vi "Auto Drive.vi"(0 "Drive Dev Ref in":T5={"DevStatus"={"status"=FALSE, "code"=0, "source"=""}, "Motors[]"=[{"DeviceStatus"={"status"=FALSE, "code"=0, "source"=""}, "Type"=enum."CAN", "PWM"={"PWM Channel"=enum."PWM 1", "DeadBand"={"Name"="", "maxPositivePwm"=0, "minPositivePwm"=0, "centerPwm"=0, "maxNegativePwm"=0, "minNegativePwm"=0, "angularRange"=0}}, "CAN"={"Device Number"=1, "SetOutput VI Ref"=variant(refnum<vi> refnum), "GetOutput VI Ref"=variant(refnum<vi> refnum), "Enable VI Ref"=variant(refnum<vi> refnum), "Disable VI Ref"=variant(refnum<vi> refnum), "Data"=variant(cluster{"Library":path, "handle":u64, "Control Mode":u16, "UsageFrame":u32, "RefNumName":string, "arbID":u32} {"Library"=path "libCTRE_PhoenixCCI.so", "handle"=21905672, "Control Mode"=0, "UsageFrame"=0, "RefNumName"="", "arbID"=33816577})}, "Invert"=TRUE, "DIO PWM"={"PWM \"Enable\" Channel"=enum."Invalid", "DIOChannel"=enum."Invalid", "PWM Rate"=0.0}}, {"DeviceStatus"={"status"=FALSE, "code"=0, "source"=""}, "Type"=enum."CAN", "PWM"={"PWM Channel"=enum."PWM 1", "DeadBand"={"Name"="", "maxPositivePwm"=0, "minPositivePwm"=0, "centerPwm"=0, "maxNegativePwm"=0, "minNegativePwm"=0, "angularRange"=0}}, "CAN"={"Device Number"=13, "SetOutput VI Ref"=variant(refnum<vi> refnum), "GetOutput VI Ref"=variant(refnum<vi> refnum), "Enable VI Ref"=variant(refnum<vi> refnum), "Disable VI Ref"=variant(refnum<vi> refnum), "Data"=variant(cluster{"Library":path, "handle":u64, "Control Mode":u16, "UsageFrame":u32, "RefNumName":string, "arbID":u32} {"Library"=path "libCTRE_PhoenixCCI.so", "handle"=21919480, "Control Mode"=0, "UsageFrame"=0, "RefNumName"="", "arbID"=33816589})}, "Invert"=FALSE, "DIO PWM"={"PWM \"Enable\" Channel"=enum."Invalid", "DIOChannel"=enum."Invalid", "PWM Rate"=0.0}}], "Square Inputs"=FALSE, "Max Output"=1.0}, 5 "Gyro Dev Ref in":T11={"DevStatus"={"status"=FALSE, "code"=0, "source"=""}, "Analog Channel"=enum."AI 1", "Gain (VoltsPerDegree/Second)"=0.0, "Gyro Type"=enum."XRS450", "Handle"=8, "SPI Bus"=enum."SPI On-Board, CS0", "Device Found"=TRUE, "Sample Rate"=2000.0, "Calibrate On Open"=FALSE, "Offset"=0.21654062499999974} {"Sample Rate" min=0.25 max=100.0 step=0.25}, 9 "Encoder Dev Ref in":T1={"DevStatus"={"status"=FALSE, "code"=0, "source"=""}, "EncoderIndex"=enum."Enc 0", "CounterIndex"=enum."Invalid", "DistancePerCount"=1.0, "Decoding Type"=enum."4x"}, 12 "X setpoint":dbl=10.0 format="%#_13g", 14 "Y setpoint":dbl=-60.0 format="%.2f") -> (4 "Drive Dev Ref out":T5={"DevStatus"={"status"=FALSE, "code"=0, "source"=""}, "Motors[]"=[{"DeviceStatus"={"status"=FALSE, "code"=0, "source"=""}, "Type"=enum."CAN", "PWM"={"PWM Channel"=enum."PWM 1", "DeadBand"={"Name"="", "maxPositivePwm"=0, "minPositivePwm"=0, "centerPwm"=0, "maxNegativePwm"=0, "minNegativePwm"=0, "angularRange"=0}}, "CAN"={"Device Number"=1, "SetOutput VI Ref"=variant(refnum<vi> refnum), "GetOutput VI Ref"=variant(refnum<vi> refnum), "Enable VI Ref"=variant(refnum<vi> refnum), "Disable VI Ref"=variant(refnum<vi> refnum), "Data"=variant(cluster{"Library":path, "handle":u64, "Control Mode":u16, "UsageFrame":u32, "RefNumName":string, "arbID":u32} {"Library"=path "libCTRE_PhoenixCCI.so", "handle"=21905672, "Control Mode"=0, "UsageFrame"=0, "RefNumName"="", "arbID"=33816577})}, "Invert"=TRUE, "DIO PWM"={"PWM \"Enable\" Channel"=enum."Invalid", "DIOChannel"=enum."Invalid", "PWM Rate"=0.0}}, {"DeviceStatus"={"status"=FALSE, "code"=0, "source"=""}, "Type"=enum."CAN", "PWM"={"PWM Channel"=enum."PWM 1", "DeadBand"={"Name"="", "maxPositivePwm"=0, "minPositivePwm"=0, "centerPwm"=0, "maxNegativePwm"=0, "minNegativePwm"=0, "angularRange"=0}}, "CAN"={"Device Number"=13, "SetOutput VI Ref"=variant(refnum<vi> refnum), "GetOutput VI Ref"=variant(refnum<vi> refnum), "Enable VI Ref"=variant(refnum<vi> refnum), "Disable VI Ref"=variant(refnum<vi> refnum), "Data"=variant(cluster{"Library":path, "handle":u64, "Control Mode":u16, "UsageFrame":u32, "RefNumName":string, "arbID":u32} {"Library"=path "libCTRE_PhoenixCCI.so", "handle"=21919480, "Control Mode"=0, "UsageFrame"=0, "RefNumName"="", "arbID"=33816589})}, "Invert"=FALSE, "DIO PWM"={"PWM \"Enable\" Channel"=enum."Invalid", "DIOChannel"=enum."Invalid", "PWM Rate"=0.0}}], "Square Inputs"=FALSE, "Max Output"=1.0}, 6 "Gyro Dev Ref out":T11={"DevStatus"={"status"=FALSE, "code"=0, "source"=""}, "Analog Channel"=enum."AI 1", "Gain (VoltsPerDegree/Second)"=0.0, "Gyro Type"=enum."XRS450", "Handle"=8, "SPI Bus"=enum."SPI On-Board, CS0", "Device Found"=TRUE, "Sample Rate"=2000.0, "Calibrate On Open"=FALSE, "Offset"=0.21654062499999974} {"Sample Rate" min=0.25 max=100.0 step=0.25}, 8 "last y value":dbl=0.16038021312985137, 10 "Encoder Dev Ref out":T1={"DevStatus"={"status"=FALSE, "code"=0, "source"=""}, "EncoderIndex"=enum."Enc 0", "CounterIndex"=enum."Invalid", "DistancePerCount"=1.0, "Decoding Type"=enum."4x"}, 15 "In Range?":bool=TRUE)   [LabVIEW 2017]
uses:
  <vilib>/Rock Robotics/WPI/RobotDrive/WPI_RobotDriveDevRef.ctl
  <vilib>/Rock Robotics/WPI/MotorControl/WPI_MotorControlDeviceRef.ctl
  <vilib>/Rock Robotics/WPI/MotorControl/WPI_MotorControlType.ctl
  <vilib>/Rock Robotics/SystemInterfaces/DIO/FPGA_DIOPWMChannel.ctl
  <vilib>/Rock Robotics/WPI/PWM/WPI_PWMDeadband.ctl
  <vilib>/Rock Robotics/SystemInterfaces/DIO/FPGA_DIOChannel.ctl
  <vilib>/Rock Robotics/WPI/Gyro/WPI_GyroDevRef.ctl
  <vilib>/Rock Robotics/SystemInterfaces/AI/FPGA_AIChannel.ctl
  <vilib>/Rock Robotics/SystemInterfaces/spilib/spi_bus.ctl
  <vilib>/Rock Robotics/WPI/Encoder/WPI_EncoderDevRef.ctl
  <vilib>/Rock Robotics/SystemInterfaces/Encoder/FPGA_EncoderIdx.ctl
  <vilib>/Rock Robotics/SystemInterfaces/Counter/FPGA_CounterCtrSystemIndex.ctl
  <vilib>/Rock Robotics/WPI/Encoder/WPI_EncoderType.ctl
  <vilib>/Rock Robotics/WPI/RobotDrive/WPI_RobotDriveArcadeDrive_Standard(NoSaturation).vi
panel:
  in  "Drive Stop Tolerance":dbl=10.0
  in  "Y Max Speed":dbl=0.8999999999999999
  in  "Slowdown Range":dbl=45.0
  in  "Turn P Multiplier":dbl=0.03
  # "turn p 0.03"
  # "degrees"
  # "x set 10"
  # "inches"
  # "y set -60.00"
  # "slowdown 60"
  # "inches"
  # "Y max 0.9"
  # "inches"
  # "Drive tol. 10"
  # "Analog"
  # "XRS"
  # "Analog"
  # "XRS"
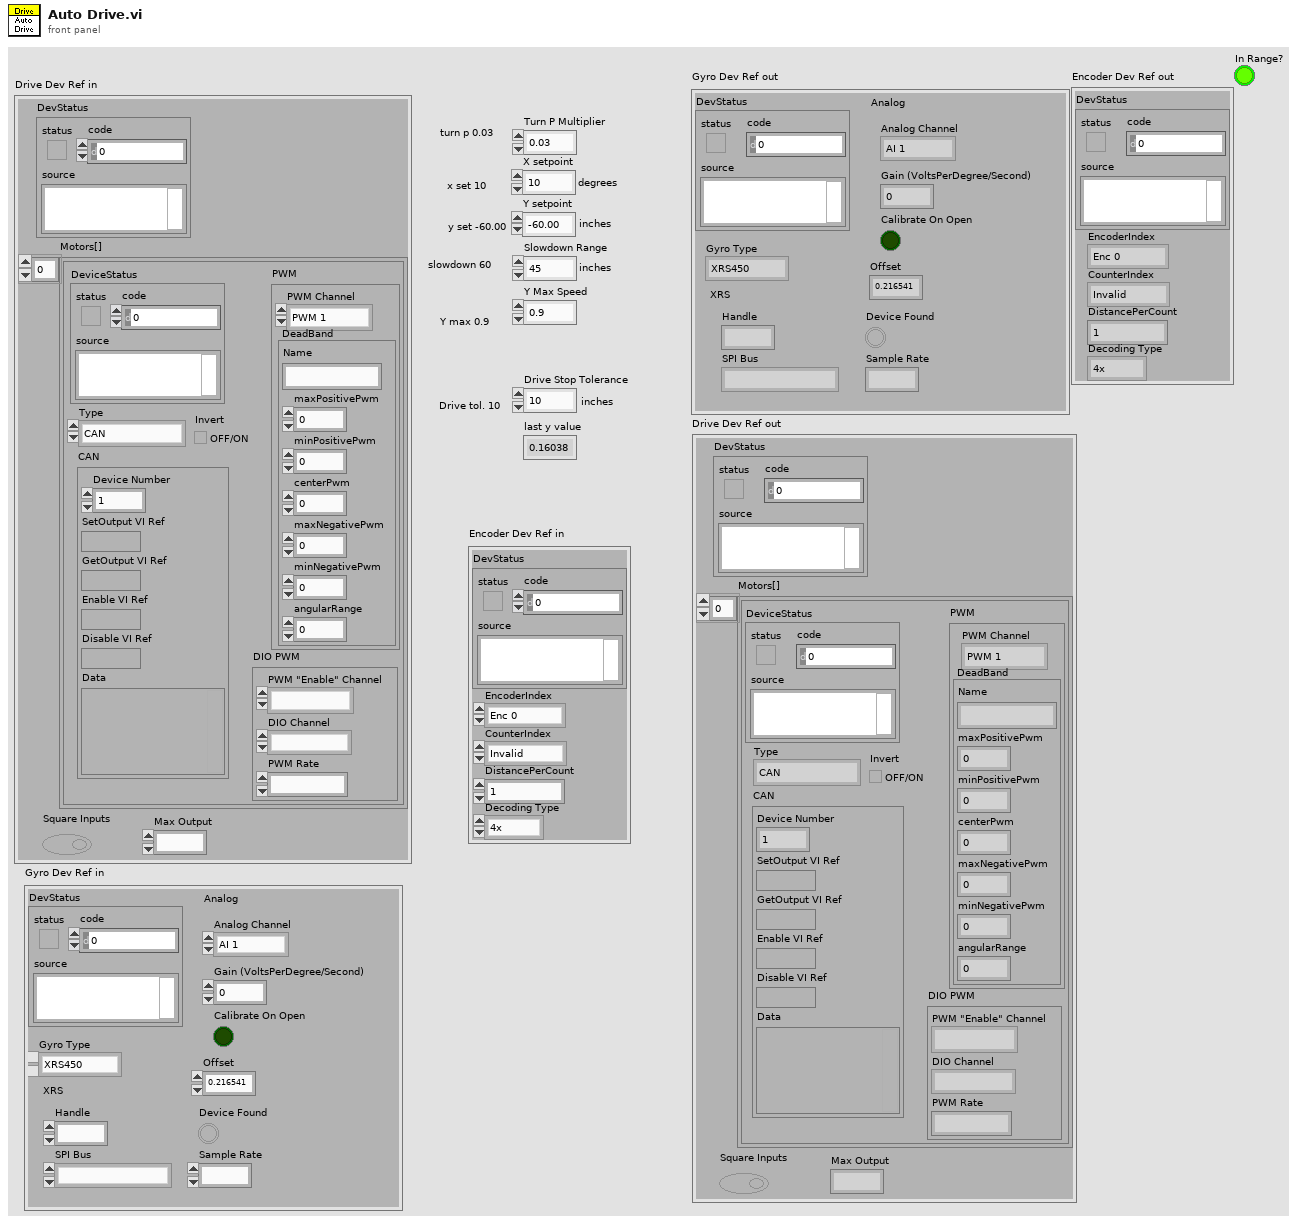
[diagram p1: front panel]
types:
  T1 = typedef "WPI_EncoderDevRef.ctl" = cluster{"DevStatus":errorcluster, "EncoderIndex":T2, "CounterIndex":T3, "DistancePerCount":dbl, "Decoding Type":T4}
  T2 = typedef "FPGA_EncoderIdx.ctl" = enum8{"Enc 0", "Enc 1", "Enc 2", "Enc 3", "Enc 4", "Enc 5", "Enc 6", "Enc 7", "Invalid"}
  T3 = typedef "FPGA_CounterCtrSystemIndex.ctl" = enum8{"Ctr 0", "Ctr 1", "Ctr 2", "Ctr 3", "Ctr 4", "Ctr 5", "Ctr 6", "Ctr 7", "Invalid"}
  T4 = typedef "WPI_EncoderType.ctl" = enum16{"1x", "2x", "4x"}
  T5 = typedef "WPI_RobotDriveDevRef.ctl" = cluster{"DevStatus":errorcluster, "Motors[]":T6[], "Square Inputs":bool, "Max Output":dbl}
  T6 = typedef "WPI_MotorControlDeviceRef.ctl" = cluster{"DeviceStatus":errorcluster, "Type":T7, "PWM":cluster{"PWM Channel":T8, "DeadBand":T9}, "CAN":cluster{"Device Number":u8, "SetOutput VI Ref":variant, "GetOutput VI Ref":variant, "Enable VI Ref":variant, "Disable VI Ref":variant, "Data":variant}, "Invert":bool, "DIO PWM":cluster{"PWM \"Enable\" Channel":T8, "DIOChannel":T10, "PWM Rate":dbl}}
  T7 = typedef "WPI_MotorControlType.ctl" = enum16{"PWM", "CAN", "DIO PWM"}
  T8 = typedef "FPGA_DIOPWMChannel.ctl" = enum8{"PWM 0", "PWM 1", "PWM 2", "PWM 3", "PWM 4", "PWM 5", "PWM 6", "PWM 7", "PWM 8", "PWM 9", "PWM MXP 0", "PWM MXP 1", "PWM MXP 2", "PWM MXP 3", "PWM MXP 4", "PWM MXP 5", "PWM MXP 6", "PWM MXP 7", "PWM MXP 8", "PWM MXP 9", "Invalid"}
  T9 = typedef "WPI_PWMDeadband.ctl" = cluster{"Name":string, "maxPositivePwm":i32, "minPositivePwm":i32, "centerPwm":i32, "maxNegativePwm":i32, "minNegativePwm":i32, "angularRange":u16}
  T10 = typedef "FPGA_DIOChannel.ctl" = enum8{"DIO 0", "DIO 1", "DIO 2", "DIO 3", "DIO 4", "DIO 5", "DIO 6", "DIO 7", "DIO 8", "DIO 9", "DIO MXP 0", "DIO MXP 1", "DIO MXP 2", "DIO MXP 3", "DIO MXP 4", "DIO MXP 5", "DIO MXP 6", "DIO MXP 7", "DIO MXP 8", "DIO MXP 9", "DIO MXP 10", "DIO MXP 11", "DIO MXP 12", "DIO MXP 13", "DIO MXP 14", "DIO MXP 15", "SPI Port CS1", "SPI Port CS2", "SPI Port CS3", "SPI Port MISO", "SPI Port MOSI", "Invalid"}
  T11 = typedef "WPI_GyroDevRef.ctl" = cluster{"DevStatus":errorcluster, "Analog Channel":T12, "Gain (VoltsPerDegree/Second)":dbl, "Gyro Type":enum16{"Analog", "XRS450"}, "Handle":i32, "SPI Bus":T13, "Device Found":bool, "Sample Rate":dbl, "Calibrate On Open":bool, "Offset":dbl}
  T12 = typedef "FPGA_AIChannel.ctl" = enum8{"AI 0", "AI 1", "AI 2", "AI 3", "AI MXP 0", "AI MXP 1", "AI MXP 2", "AI MXP 3", "Invalid"}
  T13 = typedef "spi_bus.ctl" = enum16{"SPI On-Board, CS0", "SPI On-Board, CS1", "SPI On-Board, CS2", "SPI On-Board, CS3", "SPI MXP", "Invalid"}
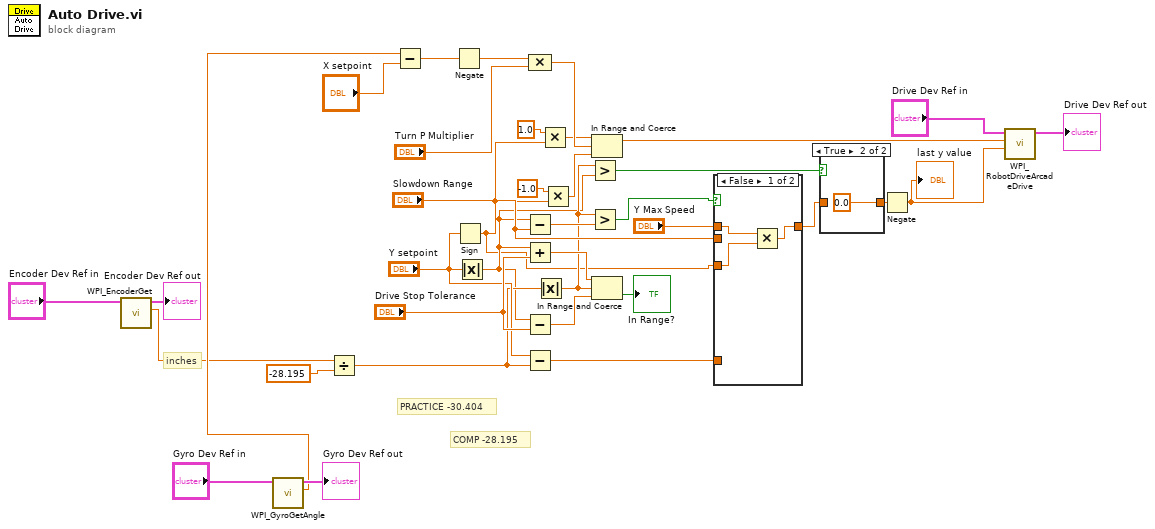
[diagram p0: block diagram]
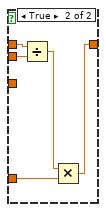
[diagram p3: hidden frame]
diagram:
  # "COMP -28.195"
  # "PRACTICE -30.404"
  # "inches"
  n1 = call <vilib>:"WPI_EncoderGet.vi"("EncoderDevRef"="Encoder Dev Ref in") -> ("Distance"=w16:dbl, "EncoderDevRef"=→"Encoder Dev Ref out":T1)  [unwired: 5 in, 4 out]
  n2 = call <vilib>:"WPI_GyroGetAngle.vi"("GyroDevRef"="Gyro Dev Ref in") -> ("Angle"=w31:dbl, "GyroDevRef"=→"Gyro Dev Ref out":T11)  [unwired: 6 in, 3 out]
  n3 = Divide(x=w16, y=-28.195) -> (x/y=w11:dbl)
  n4 = Subtract(x=w31, y="X setpoint") -> (x-y=w23:dbl)
  n5 = Negate(x=w23) -> (-x=w24:dbl)
  n6 = Sign(1:"Y setpoint") -> (0:w3:dbl)
  n7 = Absolute Value(x="Y setpoint") -> (abs(x)=w7:dbl)
  n8 = Subtract(x=w7, y="Slowdown Range") -> (x-y=w10:dbl)
  n9 = Add(x=w7, y="Drive Stop Tolerance") -> (x+y=w26:dbl)
  n10 = Subtract(x=w7, y="Drive Stop Tolerance") -> (x-y=w27:dbl)
  n11 = Subtract(x="Y setpoint", y=w11) -> (x-y=w12:dbl)
  n12 = Compound Arithmetic op=MULTIPLY(w24, "Turn P Multiplier") -> (w22:dbl)
  n13 = Absolute Value(x=w11) -> (abs(x)=w8:dbl)
  n14 = Multiply(x=1.0 ("upper limit"), y=w3) -> (x*y=w19:dbl)
  n15 = Multiply(x=-1.0 ("lower limit"), y=w3) -> (x*y=w17:dbl)
  n16 = Greater?(x=w8, y=w7) -> (0:w6:bool)
  n17 = Greater?(x=w8, y=w10) -> (0:w15:bool)
  n18 = In Range and Coerce(upper limit=w19, x=w22, lower limit=w17) -> (coerced(x)=w14:dbl)  [unwired: 1 out]
  n19 = In Range and Coerce(upper limit=w26, x=w8, lower limit=w27) -> (In Range?=→"In Range?":bool)  [unwired: 1 out]
  n20 = case shown="False" w15 {
    tunnel: [w38 w44] -> w5
    tunnel: "Y Max Speed" -> [w40 w43]
    tunnel: w12 -> [_ w45]
    tunnel: "Slowdown Range" -> [_ w42]
    tunnel: w3 -> [w39 _]
    frame False {
      n21 = Multiply(x=w40, y=w39) -> (x*y=w38:dbl)
    }
    frame True {
      n22 = Divide(x=w43, y=w42) -> (x/y=w41:dbl)
      n23 = Multiply(x=w41, y=w45) -> (x*y=w44:dbl)
    }
  }
  n24 = case shown="True" w6 {
    tunnel: w5 -> [w46 _]
    tunnel: [w46 0.0 ("Y Max Speed")] -> w4
    frame False {
    }
    frame True {
    }
  }
  n25 = Negate(x=w4) -> (-x=w2:dbl)
  "last y value" <- w2
  n26 = call-poly <vilib>:"WPI_RobotDriveArcadeDrive.vi"("Y axis value"=w2, "X axis value"=w14, "RobotDriveDevRef"="Drive Dev Ref in") -> ("RobotDriveDevRef"=→"Drive Dev Ref out":T5)  [unwired: 6 in, 2 out]
